vi "Tree_delete tag&childs.vi"(6 "tag.childs only (T)":bool=TRUE, 7 "Tree.Tag in":string, 8 "error in (no error)":errorcluster, 11 "tree RefNum in":refnum<vi>) -> (0 "error out":errorcluster, 3 "dup tree RefNum":refnum<vi>)   [LabVIEW 2014]
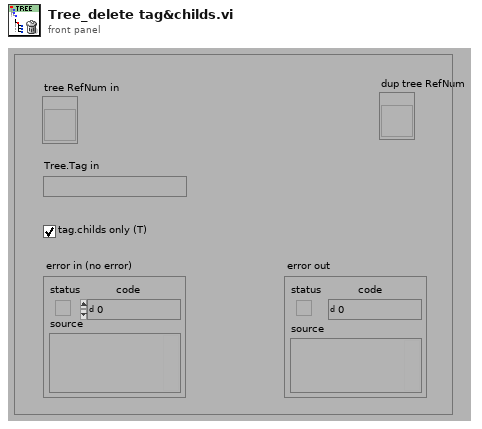
[diagram p1: front panel]
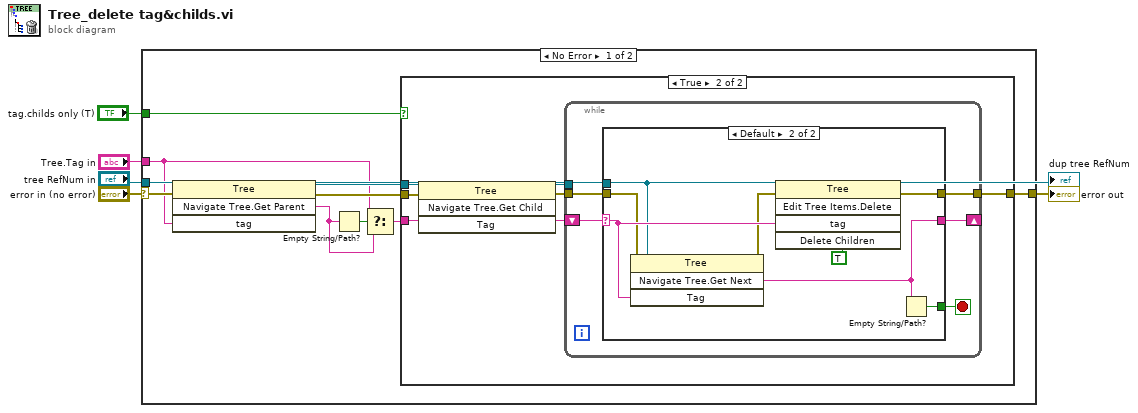
[diagram p0: block diagram]
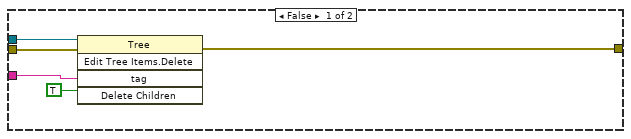
[diagram p2: hidden frame]
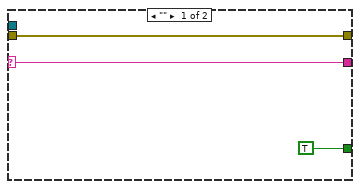
[diagram p3: hidden frame]
diagram:
  n1 = case shown="No Error" "error in (no error)" {
    selector: "error in (no error)" -> [w9 w45]
    tunnel: [w10 w45] -> w5
    tunnel: "tree RefNum in" -> [w8 _]
    tunnel: "Tree.Tag in" -> [w7 _]
    tunnel: "tag.childs only (T)" -> [w6 _]
    frame No Error {
      n2 = invoke class="Tree" method="Navigate Tree.Get Parent"(reference=w8, error in=w9, "tag"=w7) -> (reference out=w13:refnum<vi>, error out=w12:errorcluster, "Navigate Tree:Get Parent"=w14:string)  [unwired: 1 in, 1 out]
      n3 = Empty String/Path?(string/path=w14) -> (empty?=w15:bool)
      n4 = Select(t=w7, s=w15, f=w14) -> (s? t:f=w11:string)
      n5 = case shown="True" w6 {
        tunnel: w13 -> [w20 w27]
        tunnel: w12 -> [w19 w26]
        tunnel: w11 -> [w17 w25]
        tunnel: [w18 w21] -> w10
        frame False {
          n6 = invoke class="Tree" method="Edit Tree Items.Delete"(reference=w20, error in=w19, "tag"=w17, "Delete Children"=TRUE ("Delete Children?")) -> (error out=w18:errorcluster)  [unwired: 1 in, 4 out]
        }
        frame True {
          n7 = invoke class="Tree" method="Navigate Tree.Get Child"(reference=w27, error in=w26, "Tag"=w25) -> (reference out=w24:refnum<vi>, error out=w23:errorcluster, "Navigate Tree:Get Child"=w22:string)  [unwired: 1 in, 1 out]
          n8 = while {
            tunnel: w24 -> [w32]
            tunnel: w23 -> [w31]
            shift-right: [w29] -> _
            shift-left: w22 -> [w30]
            tunnel: [w28] -> w21
            stop <- w33 stop-if-true
            n9 = case shown="Default" w30 {
              selector: w30 -> [w35 w43]
              tunnel: w32 -> [_ w40]
              tunnel: w31 -> [w34 w41]
              tunnel: [TRUE w38] -> w33
              tunnel: [w35 w39] -> w29
              tunnel: [w34 w37] -> w28
              frame "" {
              }
              frame Default {
                n10 = invoke class="Tree" method="Navigate Tree.Get Next"(reference=w40, error in=w41, "Tag"=w43) -> (error out=w42:errorcluster, "Navigate Tree:Get Next Item"=w39:string)  [unwired: 1 in, 2 out]
                n11 = invoke class="Tree" method="Edit Tree Items.Delete"(reference=w40, error in=w42, "tag"=w43, "Delete Children"=TRUE ("Delete Children?")) -> (error out=w37:errorcluster)  [unwired: 1 in, 4 out]
                n12 = Empty String/Path?(string/path=w39) -> (empty?=w38:bool)
              }
            }
          }
        }
      }
    }
    frame Error {
    }
  }
  "error out" <- w5
  "dup tree RefNum" <- "tree RefNum in"
